vi "BRig_dataMTrig_init_setDefault.vi"(11 "input_dataMTrig":u16[](array[numeric])) -> (3 "output_dataMTrig":u16[](array[numeric]))   [LabVIEW 2014]
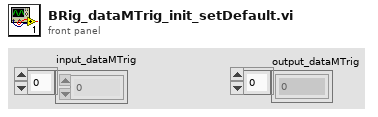
[diagram p1: front panel]
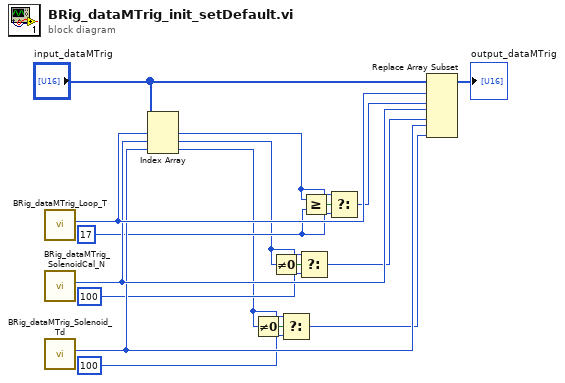
[diagram p0: block diagram]
diagram:
  w5 = u16 17 ("new element/subarray")
  n1 = call "BRig_dataMTrig_Loop_T.vi"() -> ("output_Loop_T"=w14:i32)  [unwired: 11 in]
  n2 = call "BRig_dataMTrig_SolenoidCal_N.vi"() -> ("output_SolenoidCal_N"=w11:i32)  [unwired: 11 in]
  n3 = call "BRig_dataMTrig_Solenoid_Td.vi"() -> ("output_Solenoid_Td"=w8:i32)  [unwired: 11 in]
  n4 = Index Array(array="input_dataMTrig", index #1=w14, index #2=w11, index #3=w8) -> (element #1=w6:u16, element #2=w4:u16, element #3=w2:u16)
  n5 = Not Equal To 0?(x=w2) -> (x != 0?=w9:bool)
  n6 = Not Equal To 0?(x=w4) -> (x != 0?=w12:bool)
  n7 = Select(t=w2, s=w9, f=u16 100 ("new element/subarray")) -> (s? t:f=w7:u16)
  n8 = Select(t=w4, s=w12, f=u16 100 ("new element/subarray")) -> (s? t:f=w10:u16)
  n9 = Greater Or Equal?(x=w6, y=w5) -> (x >= y?=w15:bool)
  n10 = Select(t=w6, s=w15, f=w5) -> (s? t:f=w13:u16)
  n11 = Replace Array Subset(array="input_dataMTrig", new element #1=w13, index #1=w14, new element #2=w10, index #2=w11, new element #3=w7, index #3=w8) -> (→"output_dataMTrig":u16[])
